vi "Set Speaker Lighting.vi"(8 "error in (no error)":errorcluster, 10 "Lighting Zone":T1=enum."Rear right", 11 "LED Color":u32(colorbox)) -> (0 "error out":errorcluster)   [LabVIEW 2025, in "Logitech Devices.lvlib"]
uses:
  Logitech Devices.lvlib
  TypeDefs/Speaker Lighting Zones.ctl
  <vilib>/Utility/colorconv.llb/Color to RGB.vi
  <vilib>/Utility/error.llb/Error Cluster From Error Code.vi
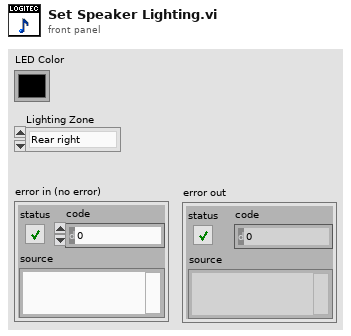
[diagram p1: front panel]
types:
  T1 = typedef "Logitech Devices.lvlib/Speaker Lighting Zones.ctl" = enum8{"Front left", "Front right", "Rear left", "Rear right"}
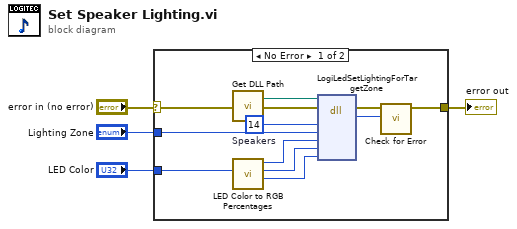
[diagram p0: block diagram]
diagram:
  n1 = case shown="No Error" "error in (no error)" {
    selector: "error in (no error)" -> [w15 w16]
    tunnel: [w7 w16] -> w3
    tunnel: "Lighting Zone" -> [w9 _]
    tunnel: "LED Color" -> [w13 _]
    frame No Error {
      w6 = u8 14  # Speakers
      n2 = call "Get DLL Path.vi"() -> ("LG Hub SDK DLL"=w5:path)  [unwired: 3 in]
      n3 = call "LED Color to RGB Percentages.vi"("LED Color"=w13) -> ("Blue %"=w10:u8, "Green %"=w11:u8, "Red %"=w12:u8)  [unwired: 8 in]
      n4 = dll-call lib="C:/Program Files/LGHUB/sdks/sdk_legacy_led_x86.dll" fn="LogiLedSetLightingForTargetZone"(path in=w5, error in=w15, "Device Type"=w6, "Zone"=w9, "Red Percentage"=w12, "Green Percentage"=w11, "Blue Percentage"=w10) -> (error out=w8:errorcluster, "return type"=w14:u8)  [unwired: 6 in, 1 out]
      n5 = call "Check for Error.vi"("DLL-call return value"=w14, "error in (no error)"=w8) -> ("error out"=w7:errorcluster)  [unwired: 9 in]
    }
    frame Error {
    }
  }
  "error out" <- w3
